vi "Configure HSDIO_PFI Channels.vi"(10 "Pins":string[](array[string])=["SW1", "SW2"], 11 "Semiconductor Module Context":T1) -> (0 "error out":errorcluster)   [LabVIEW 2013]
uses:
  <vilib>/NI_TestStand_SemiconductorModule/NI_TestStand_Semiconductor_Module.lvlibp/PinMap/General/SemiconductorModuleContext.ctl
  <vilib>/NI_TestStand_SemiconductorModule/NI_TestStand_Semiconductor_Module.lvlibp/PinMap/HSDIO/PinsToNIHSDIOSessions.vi
  <vilib>/NI_TestStand_SemiconductorModule/NI_TestStand_Semiconductor_Module.lvlibp
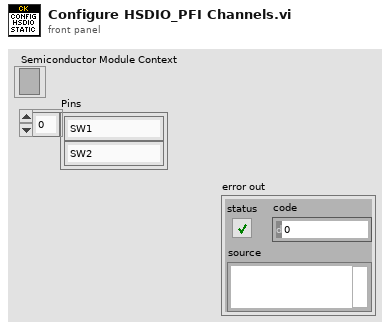
[diagram p1: front panel]
types:
  T1 = typedef "NI_TestStand_Semiconductor_Module.lvlibp/SemiconductorModuleContext.ctl" = refnum<k7>
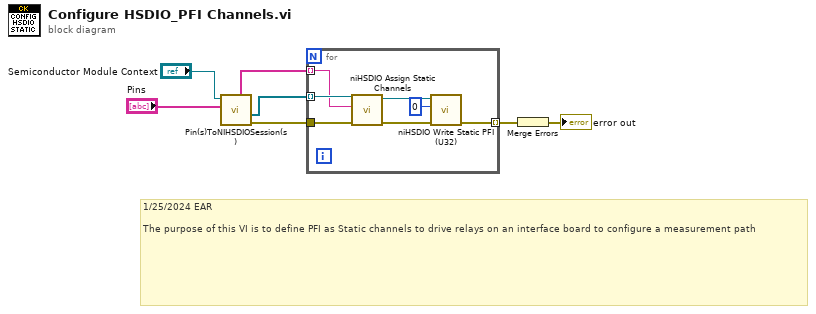
[diagram p0: block diagram]
diagram:
  # "1/25/2024 EAR\n\nThe purpose of this VI is to define PFI as Static channels to drive relays on an interface board to configure a measurement path"
  n1 = call-poly <vilib>:"Pin(s)ToNIHSDIOSession(s).vi"("Pins"="Pins", "Semiconductor Module Context"="Semiconductor Module Context") -> ("error out"=w4:errorcluster, "Generation Sessions"=w6:refnum<k15>[], "Channel Lists"=w7:string[])  [unwired: 4 in, 3 out]
  n2 = for {
    tunnel: w7 -> [w9] mode=indexing
    tunnel: w6 -> [w14] mode=indexing
    tunnel: w4 -> [w13]
    tunnel: [w11] -> w2 mode=indexing
    n3 = call <instrlib>:"niHSDIO Assign Static Channels.vi"("error in (no error)"=w13, "channel list (all:\"\")"=w9, "instrument handle"=w14) -> ("error out"=w12:errorcluster, "instrument handle out"=w10:refnum<k15>)  [unwired: 7 in]
    n4 = call <instrlib>:"niHSDIO Write Static PFI (U32).vi"("error in (no error)"=w12, "write data (0x0000)"=u32 0, "instrument handle"=w10) -> ("error out"=w11:errorcluster)  [unwired: 7 in, 1 out]
  }
  n5 = Merge Errors(w2) -> (→"error out":errorcluster)
